vi "Initialize RF Sessions.vi"(0 "RF Subsystem Session Provider in":refnum<class "RF Subsystem Session Provider.lvclass">, 5 "TSM Context":T1, 11 "error in":errorcluster) -> (4 "RF Subsystem Session Provider out":refnum<class "RF Subsystem Session Provider.lvclass">, 15 "error out":errorcluster)   [LabVIEW 2023, in "RFFixtureCharact.PXI.lvlib" / "RF Subsystem Session Provider.lvclass"]
uses:
  RF Subsystem Session Provider.lvclass
  <vilib>/NI_TestStand_SemiconductorModule/NI_TestStand_Semiconductor_Module.lvlibp/PinMap/General/SemiconductorModuleContext.ctl
  Common/RF Subsystem Session Provider/Utilities/Global Data Id Prefix.vi
  <vilib>/NI_TestStand_SemiconductorModule/NI_TestStand_Semiconductor_Module.lvlibp/PinMap/Site and Global Data/SetGlobalData.vi
  RF Subsystem Session Provider.lvclass/RF Subsystem Session Provider.ctl
  <vilib>/NI_TestStand_SemiconductorModule/NI_TestStand_Semiconductor_Module.lvlibp
  Common/RFCalAndFixtureCharact.Common.lvlib
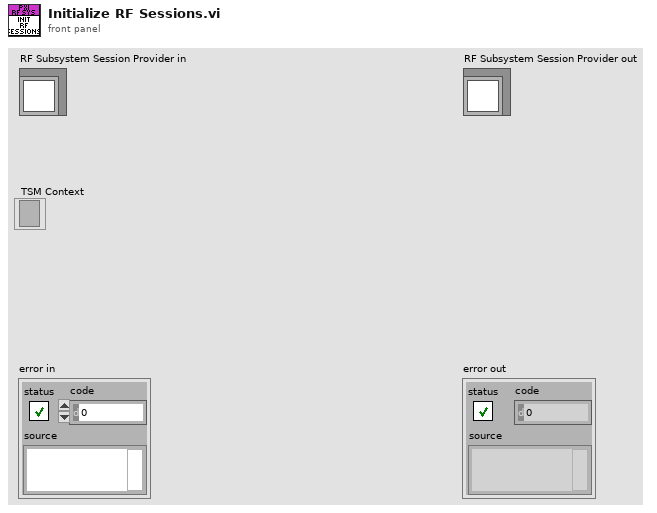
[diagram p1: front panel]
types:
  T1 = typedef "NI_TestStand_Semiconductor_Module.lvlibp/SemiconductorModuleContext.ctl" = refnum<k7>
  T2 = enum16{"OnboardClock", "RefIn", "PXI_Clk", "ClkIn", "RefIn2", "PXI_ClkMaster"}
  T3 = typedef "NI_TestStand_Semiconductor_Module.lvlibp/ModelBasedInstrumentInstanceData.ctl" = cluster{"Instrument Name":string, "Instrument Model":string}
  T4 = typedef "NI_TestStand_Semiconductor_Module.lvlibp/ModelBasedResourcePropertyList.ctl" = cluster{"Instrument Resource":string, "Properties":T5[]}
  T5 = typedef "NI_TestStand_Semiconductor_Module.lvlibp/ModelBasedInstrumentProperty.ctl" = cluster{"Property Name":string, "Property Value":string}
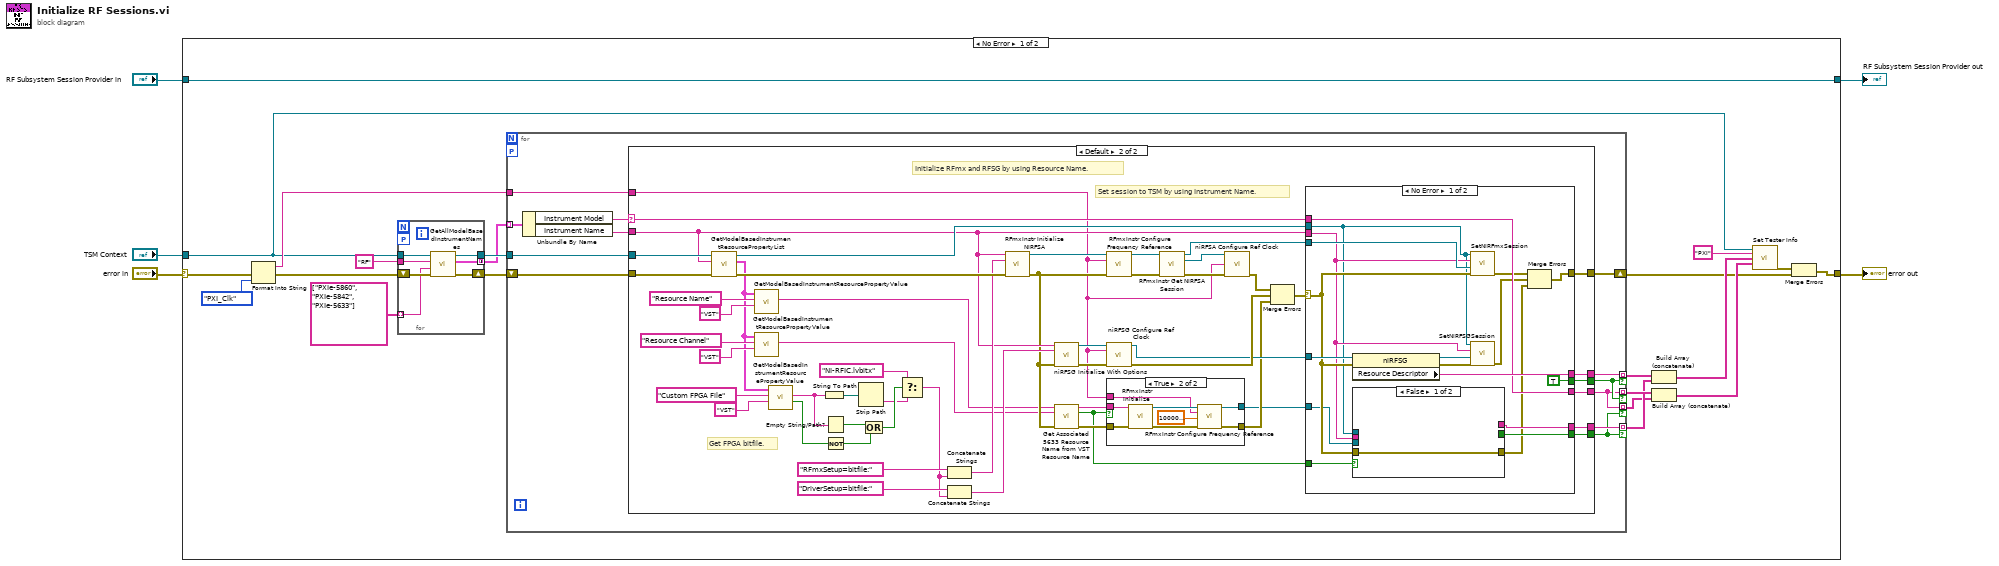
[diagram p0: block diagram]
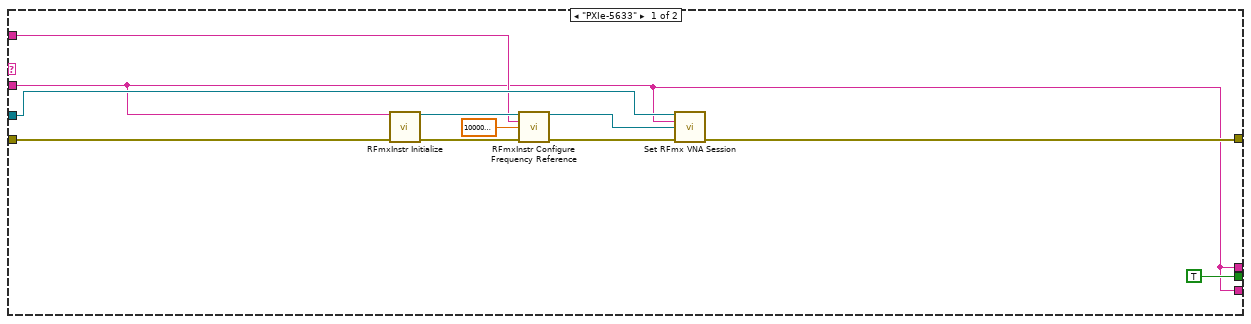
[diagram p2: hidden frame]
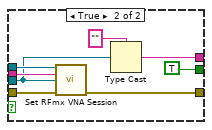
[diagram p4: hidden frame]
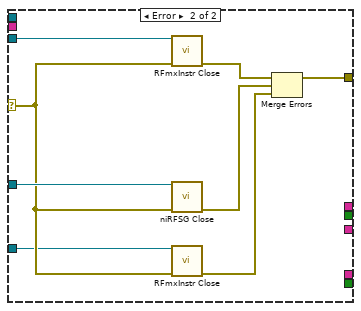
[diagram p5: hidden frame]
diagram:
  n1 = case shown="No Error" "error in" {
    selector: "error in" -> [w25 w155]
    tunnel: [w18 w155] -> w1
    tunnel: "TSM Context" -> [w16 _]
    tunnel: "RF Subsystem Session Provider in" -> [w26 w154]
    tunnel: [w26 w154] -> w2
    frame No Error {
      n2 = Format Into String(error in=w25, T2."PXI_Clk" ("Reference Clock Source In")) -> (resulting string=w23:string, error out=w15:errorcluster)  [unwired: 2 in]
      n3 = for {
        shift-right: [w30] -> w9
        shift-left: w15 -> [w32]
        tunnel: "RF" ("Category") -> [w29]
        tunnel: w16 -> [w33]
        tunnel: [w31] -> w10
        workers-P: _ -> [_]
        tunnel: [w28] -> w7 mode=concatenating
        tunnel: string[] ["PXIe-5860", "PXIe-5842", "PXIe-5633"] -> [w27] mode=indexing
        n4 = call <vilib>:"GetAllModelBasedInstrumentNames.vi"("error in (no error)"=w32, "Subcategory"=w27, "Category"=w29, "Semiconductor Module Context"=w33) -> ("error out"=w30:errorcluster, "Model-Based Instruments"=w28:T3[], "Semiconductor Module Context Out"=w31:T1)  [unwired: 5 in]
      }
      n5 = for {
        tunnel: w7 -> [w45] mode=indexing
        shift-right: [w40] -> w17
        shift-left: w9 -> [w42]
        workers-P: _ -> [_]
        tunnel: w10 -> [w44]
        tunnel: w23 -> [w43]
        tunnel: [w41] -> w14 mode=indexing if=w38
        tunnel: [w36] -> w13 mode=indexing if=w38
        tunnel: [w37] -> w12 mode=indexing if=w35
        tunnel: [w36] -> w11 mode=indexing if=w35
        n6 = Unbundle By Name(w45) -> ("Instrument Model"=w34:string, "Instrument Name"=w39:string)
        n7 = case shown="Default" w34 {
          selector: w34 -> [_ w58]
          tunnel: w44 -> [w50 w90]
          tunnel: w43 -> [w49 w57]
          tunnel: w42 -> [w51 w83]
          tunnel: [w46 w79] -> w41
          tunnel: [w48 w77] -> w40
          tunnel: w39 -> [w46 w76]
          tunnel: [TRUE w75] -> w38
          tunnel: [_ w68] -> w37
          tunnel: [w46 w67] -> w36
          tunnel: [_ w66] -> w35
          frame "PXIe-5633" {
            n8 = call <vilib>:"RFmxInstr Initialize.vi"("Resource Name"=w46, "error in (no error)"=w51) -> ("Instrument Handle Out"=w56:refnum<k21>, "error out"=w54:errorcluster)  [unwired: 11 in, 1 out]
            n9 = call <vilib>:"RFmxInstr Configure Frequency Reference.vi"("Instrument Handle In"=w56, "Frequency Reference Source"=w49, "Frequency (Hz)"=100000000.0 ("clock rate"), "error in (no error)"=w54) -> ("Instrument Handle Out"=w52:refnum<k21>, "error out"=w53:errorcluster)  [unwired: 10 in]
            n10 = call "Set RFmx VNA Session.vi"("TSM Context"=w50, "VST Instrument Name"=w46, "RFmx VNA Session"=w52, "error in"=w53) -> ("error out"=w48:errorcluster)  [unwired: 11 in]
          }
          frame Default {
            # "Set session to TSM by using Instrument Name."
            # "Initialize RFmx and RFSG by using Resource Name."
            # "Get FPGA bitfile."
            n11 = call <vilib>:"GetModelBasedInstrumentResourcePropertyList.vi"("error in (no error)"=w83, "Instrument Name"=w76, "Semiconductor Module Context"=w90) -> ("error out"=w99:errorcluster, "Model-Based Instrument Resource Property List"=w61:T4[], "Semiconductor Module Context Out"=w81:T1)  [unwired: 6 in]
            n12 = call <vilib>:"GetModelBasedInstrumentResourcePropertyValue.vi"("Resource Name"="VST", "Property Name"="Resource Name", "Model-Based Instrument Resource Property List"=w61) -> ("Property Value"=w60:string)  [unwired: 6 in, 2 out]
            n13 = call <vilib>:"GetModelBasedInstrumentResourcePropertyValue.vi"("Resource Name"="VST", "Property Name"="Resource Channel", "Model-Based Instrument Resource Property List"=w61) -> ("Property Value"=w59:string)  [unwired: 6 in, 2 out]
            n14 = call <vilib>:"GetModelBasedInstrumentResourcePropertyValue.vi"("Resource Name"="VST", "Property Name"="Custom FPGA File", "Model-Based Instrument Resource Property List"=w61) -> ("Is Found"=w104:bool, "Property Value"=w92:string)  [unwired: 6 in, 1 out]
            n15 = String To Path(string=w92) -> (path=w98:path)
            n16 = Empty String/Path?(string/path=w92) -> (empty?=w103:bool)
            n17 = Not(x=w104) -> (.not. x?=w105:bool)
            n18 = Strip Path(path=w98) -> (name=w91:string)  [unwired: 1 out]
            n19 = Or(x=w103, y=w105) -> (x .or. y?=w106:bool)
            n20 = Select(t="NI-RFIC.lvbitx", s=w106, f=w91) -> (s? t:f=w94:string)
            n21 = Concatenate Strings("RFmxSetup=bitfile:" ("format string"), w94) -> (w96:string)
            n22 = Concatenate Strings("DriverSetup=bitfile:" ("option string"), w94) -> (w93:string)
            n23 = call <vilib>:"RFmxInstr Initialize NIRFSA.vi"("Resource Name"=w76, "Option String"=w96, "error in (no error)"=w99) -> ("Instrument Handle Out"=w109:refnum<k21>, "error out"=w72:errorcluster)  [unwired: 10 in, 1 out]
            n24 = call <instrlib>:"niRFSG Initialize With Options.vi"("resource name"=w76, "option string"=w93, "error in"=w72) -> ("instrument handle"=w108:refnum<k15>, "error out"=w107:errorcluster)  [unwired: 11 in]
            n25 = call "Get Associated 5633 Resource Name from VST Resource Name.vi"("VST Instrument Name"=w60, "VST Channel"=w59, "error in"=w72) -> ("5633 Resource Name"=w73:string, "Found"=w70:bool, "error out"=w74:errorcluster)  [unwired: 10 in]
            n26 = call <vilib>:"RFmxInstr Configure Frequency Reference.vi"("Instrument Handle In"=w109, "Frequency Reference Source"=w57, "error in (no error)"=w72) -> ("Instrument Handle Out"=w85:refnum<k21>, "error out"=w84:errorcluster)  [unwired: 11 in]
            n27 = call <instrlib>:"niRFSG Configure Ref Clock.vi"("instrument handle"=w108, "ref clock source"=w57, "error in"=w107) -> ("instrument handle out"=w78:refnum<k15>, "error out"=w86:errorcluster)  [unwired: 11 in]
            n28 = case shown="True" w70 {
              tunnel: w74 -> [w110 w118]
              tunnel: w73 -> [_ w117]
              tunnel: [_ w113] -> w69
              tunnel: [w110 w114] -> w71
              tunnel: w57 -> [_ w111]
              frame False {
              }
              frame True {
                n29 = call <vilib>:"RFmxInstr Initialize.vi"("Resource Name"=w117, "error in (no error)"=w118) -> ("Instrument Handle Out"=w116:refnum<k21>, "error out"=w115:errorcluster)  [unwired: 11 in, 1 out]
                n30 = call <vilib>:"RFmxInstr Configure Frequency Reference.vi"("Instrument Handle In"=w116, "Frequency Reference Source"=w111, "Frequency (Hz)"=100000000.0 ("clock rate"), "error in (no error)"=w115) -> ("Instrument Handle Out"=w113:refnum<k21>, "error out"=w114:errorcluster)  [unwired: 10 in]
              }
            }
            n31 = call <vilib>:"RFmxInstr Get NIRFSA Session.vi"("Instrument Handle In"=w85, "error in (no error)"=w84) -> ("Instrument Handle Out"=w80:refnum<k21>, "NI RFSA Session"=w88:refnum<k15>, "error out"=w89:errorcluster)  [unwired: 11 in]
            n32 = call <instrlib>:"niRFSA Configure Ref Clock.vi"("instrument handle"=w88, "clock source"=w57, "error in"=w89) -> ("error out"=w87:errorcluster)  [unwired: 11 in, 1 out]
            n33 = Merge Errors(w87, w86, w71) -> (w82:errorcluster)
            n34 = case shown="No Error" w82 {
              selector: w82 -> [w129 w148]
              tunnel: [w119 w149] -> w77
              tunnel: w81 -> [w125 _]
              tunnel: w78 -> [w135 w153]
              tunnel: w76 -> [w127 _]
              tunnel: w80 -> [w136 w151]
              tunnel: [TRUE _] -> w75
              tunnel: [w131 _] -> w79
              tunnel: w58 -> [w130 _]
              tunnel: [w130 _] -> w67
              tunnel: w70 -> [w128 _]
              tunnel: w69 -> [w126 w147]
              tunnel: [w124 _] -> w68
              tunnel: [w123 _] -> w66
              frame No Error {
                n35 = property class="niRFSG"(reference=w135, error in=w129) -> (reference out=w134:refnum<k15>, error out=w133:errorcluster, "Resource Descriptor"=w131:string)
                n36 = case shown="False" w128 {
                  tunnel: w125 -> [_ w145]
                  tunnel: w127 -> [_ w144]
                  tunnel: w129 -> [w137 w143]
                  tunnel: w126 -> [_ w139]
                  tunnel: [w137 w141] -> w120
                  tunnel: [_ w140] -> w124
                  tunnel: [_ TRUE] -> w123
                  frame False {
                  }
                  frame True {
                    n37 = call "Set RFmx VNA Session.vi"("TSM Context"=w145, "VST Instrument Name"=w144, "RFmx VNA Session"=w139, "error in"=w143) -> ("error out"=w141:errorcluster)  [unwired: 11 in]
                    n38 = Type Cast(type="", x=w139) -> (*(type *) &x=w140:string)
                  }
                }
                n39 = call <vilib>:"SetNIRFmxSession.vi"("error in (no error)"=w129, "NI-RFmx Session"=w136, "Instrument Name"=w127, "Semiconductor Module Context"=w125) -> ("error out"=w122:errorcluster)  [unwired: 6 in, 1 out]
                n40 = call <vilib>:"SetNIRFSGSession.vi"("error in (no error)"=w133, "NI-RFSG Session"=w134, "Instrument Name"=w127, "Semiconductor Module Context"=w125) -> ("error out"=w121:errorcluster)  [unwired: 6 in, 1 out]
                n41 = Merge Errors(w122, w121, w120) -> (w119:errorcluster)
              }
              frame Error {
                n42 = call <vilib>:"RFmxInstr Close.vi"("Instrument Handle In"=w151, "error in (no error)"=w148) -> ("error out"=w152:errorcluster)  [unwired: 13 in]
                n43 = call <instrlib>:"niRFSG Close.vi"("instrument handle"=w153, "error in"=w148) -> ("error out"=w150:errorcluster)  [unwired: 13 in]
                n44 = call <vilib>:"RFmxInstr Close.vi"("Instrument Handle In"=w147, "error in (no error)"=w148) -> ("error out"=w146:errorcluster)  [unwired: 13 in]
                n45 = Merge Errors(w152, w150, w146) -> (w149:errorcluster)
              }
            }
          }
        }
      }
      n46 = Build Array (concatenate)(w14, w12) -> (w21:string[])
      n47 = Build Array (concatenate)(w13, w11) -> (w20:string[])
      n48 = call "Set Tester Info.vi"("TSM Context In"=w16, "Tester Type"="PXI", "Resource Descriptors"=w21, "Instrument Models"=w20) -> ("error out"=w19:errorcluster)  [unwired: 10 in, 1 out]
      n49 = Merge Errors(w19, w17) -> (w18:errorcluster)
    }
    frame Error {
    }
  }
  "error out" <- w1
  "RF Subsystem Session Provider out" <- w2
